vi "Module Init.vi"(8 "error in (no error)":errorcluster, 11 "TestModule in":refnum<class "TestModule.lvclass">) -> (0 "error out":errorcluster, 3 "TestModule out":refnum<class "TestModule.lvclass">)   [LabVIEW 2020, in "VolatusScratch.lvlib" / "TestModule.lvclass"]
uses:
  TestModule.lvclass
  C:/dev/lv20CE/relink/lv-volatus/Volatus/Module/Module.lvclass
  TestModule.lvclass/TestModule.ctl
  Volatus/Module/Module.lvclass
  C:/dev/lv20CE/relink/lv-volatus/VolatusScratch/TestModule/TestModule.lvclass
  VolatusConfig/Task/Task.lvclass
  lv-vecto/Vecto/Group/Group.lvclass
  C:/dev/lv20CE/relink/lv-vecto/Vecto/GroupAbstract/GroupAbstract.lvclass
  C:/dev/lv20CE/relink/lv-vecto/Vecto/Group/Group.lvclass
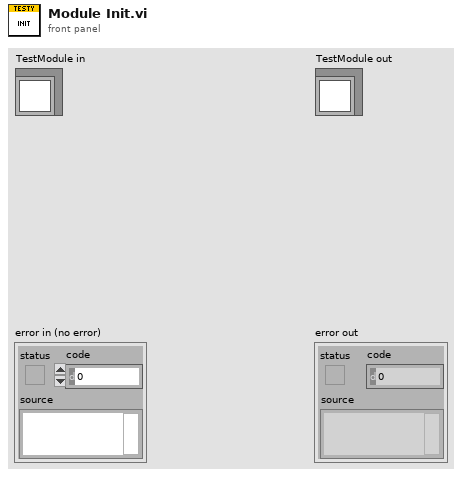
[diagram p1: front panel]
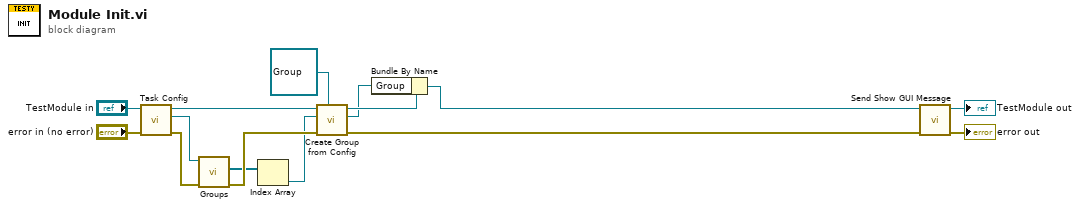
[diagram p0: block diagram]
diagram:
  n1 = call "Task Config.vi"("error in (no error)"="error in (no error)", "Module in"="TestModule in") -> ("error out"=w8:errorcluster, "Task Config"=w9:refnum<class "Task.lvclass">, "Module out"=w11:refnum<class "TestModule.lvclass">)  [unwired: 7 in]
  n2 = call "Groups.vi"("error in (no error)"=w8, "Task in"=w9) -> ("error out"=w15:errorcluster, "Groups"=w7:refnum<class "Group.lvclass">[])  [unwired: 7 in, 1 out]
  n3 = Index Array(array=w7) -> (element=w5:refnum<class "Group.lvclass">)  [unwired: 1 in]
  n4 = call "Create Group from Config.vi"("Group Type (Abstract)"=refnum<class "Group.lvclass"> refnum ("Vecto.lvlib:Group.lvclass"), "error in (no error)"=w15, "Group Config"=w5, "Module in"=w11) -> ("error out"=w1:errorcluster, "Group"=w2:refnum<class "Group.lvclass">, "Module out"=w6:refnum<class "TestModule.lvclass">)  [unwired: 5 in]
  n5 = Bundle By Name(cluster=w6, "Group"=w2) -> (w3:refnum<class "TestModule.lvclass">)
  n6 = call "Send Show GUI Message.vi"("error in (no error)"=w1, "Module in"=w3) -> ("error out"=→"error out":errorcluster, "Module out"=→"TestModule out":refnum<class "TestModule.lvclass">)  [unwired: 8 in]
